vi "lfield_acq_single_frame.vi"(8 "error in (no error)":errorcluster, 11 "lightfield_class in":refnum<class "lightfield_class.lvclass">) -> (0 "error out":errorcluster, 2 "image_data":T1, 3 "lightfield_class out":refnum<class "lightfield_class.lvclass">)   [LabVIEW 2015, in "lightfield_class.lvclass"]
uses:
  lightfield_class.lvclass
  lightfield_class.lvclass/lightfield_class.ctl
  lightfield-automation-labview/LightField Automation.lvclass
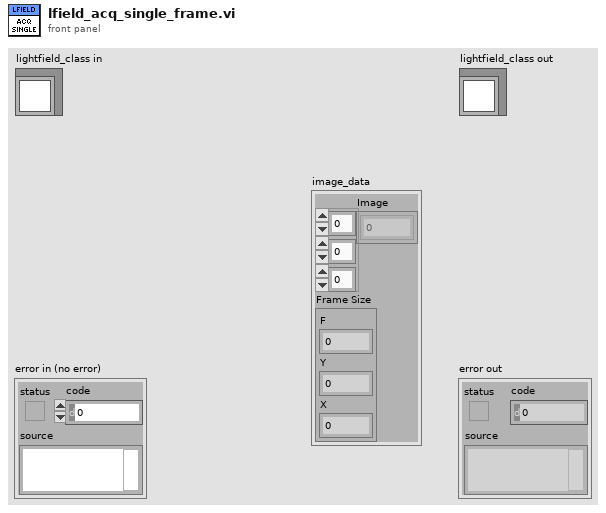
[diagram p1: front panel]
types:
  T1 = cluster{"Image":dbl[][][], "Frame Size":cluster{"F":i32, "Y":i32, "X":i32}}
  T2 = cluster{"Image":dbl[][][], "Frame Size":cluster{"F":i32, "Y":i32, "X":i32}}[]
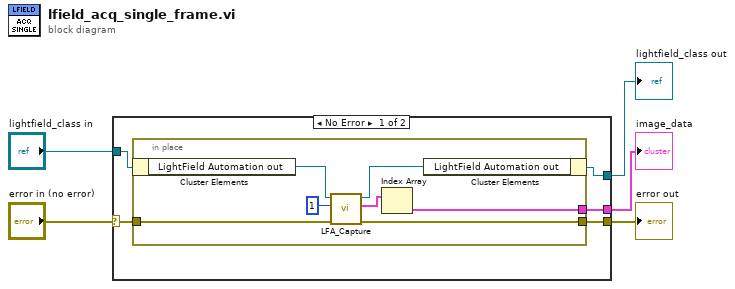
[diagram p0: block diagram]
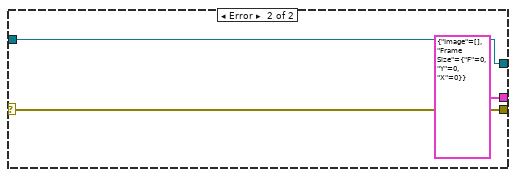
[diagram p2: hidden frame]
diagram:
  n1 = case shown="No Error" "error in (no error)" {
    selector: "error in (no error)" -> [w9 w20]
    tunnel: [w8 w20] -> w4
    tunnel: [w7 w19] -> w2
    tunnel: "lightfield_class in" -> [w10 w19]
    tunnel: [w6 T1 {"Image"=[], "Frame Size"={"F"=0, "Y"=0, "X"=0}} ("Cluster")] -> w1
    frame No Error {
      n2 = in-place {
        in-place-border: w9 -> [w16]
        in-place-border: [w12] -> w8
        in-place-border: [w11] -> w6
        n3 = in-place-cluster #1(w10) -> ("LightField Automation out"=w17:refnum<class "LightField Automation.lvclass">)
        n4 = call "LFA_Capture.vi"("error in (no error)"=w16, "Frames"=1, "LightField Automation in"=w17) -> ("error out"=w12:errorcluster, "Data"=w15:T2, "LightField Automation out"=w14:refnum<class "LightField Automation.lvclass">)  [unwired: 6 in]
        n5 = Index Array(array=w15) -> (element=w11:T1)  [unwired: 1 in]
        n6 = in-place-cluster #1("LightField Automation out"=w14) -> (w7:refnum<class "lightfield_class.lvclass">)
      }
    }
    frame Error {
    }
  }
  "error out" <- w4
  "lightfield_class out" <- w2
  "image_data" <- w1
